vi "Tree_ShowScrollBar.vi"(8 "error in (no error)":errorcluster, 11 "Tree":refnum<vi>) -> (0 "error out":errorcluster)   [LabVIEW 2017]
doc: "Determine, based on the contents of a tree control, whether or not to display its vertical and horizontal scrollbars."
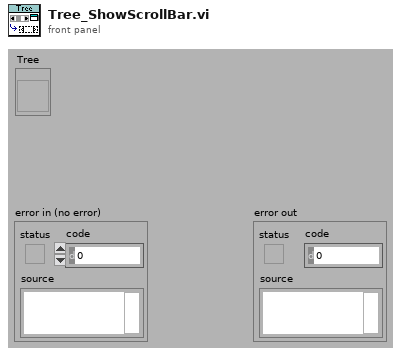
[diagram p1: front panel]
types:
  T1 = enum16{"User-specified Font", "Application Font", "System Font", "Dialog Font"}
  T2 = typedef "LVNodeAndColumnTypeDef.ctl" = cluster{"Node":string, "Column":i32}
  T3 = cluster{"left":i16, "top":i16, "right":i16, "bottom":i16}
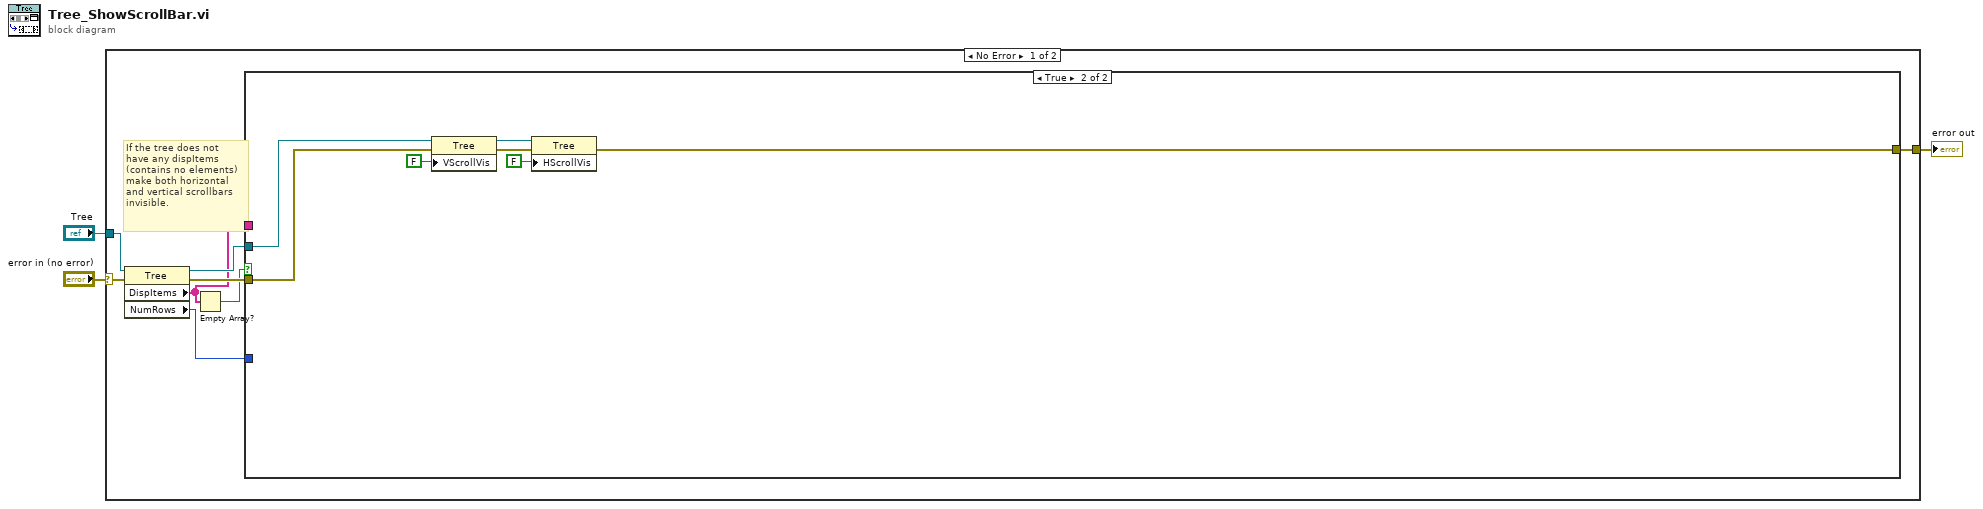
[diagram p0: block diagram]
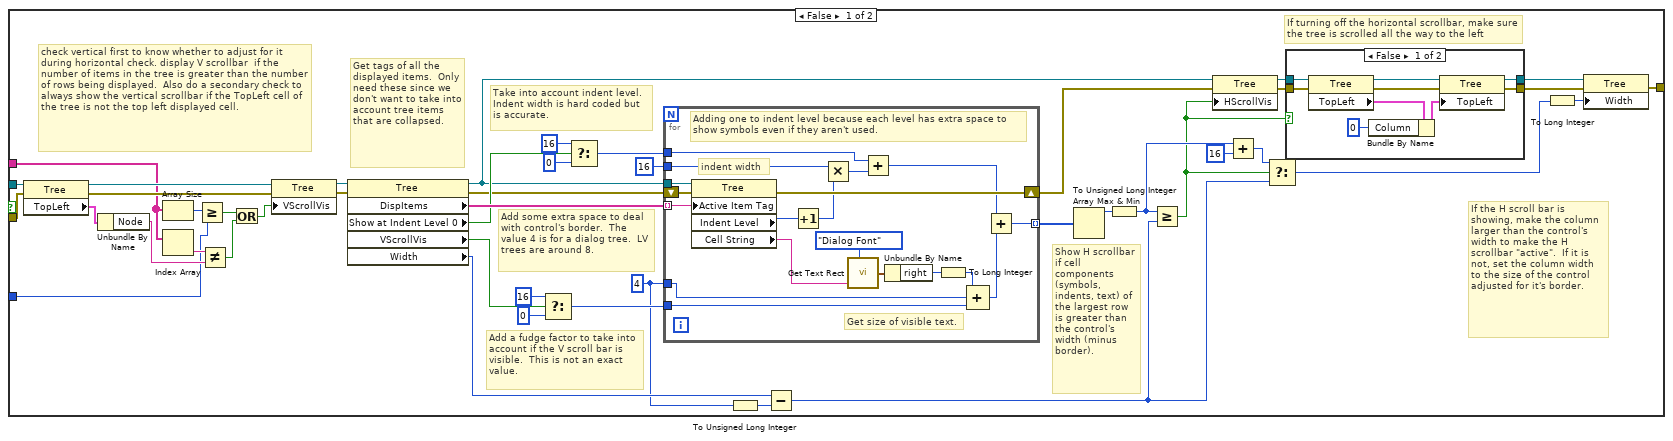
[diagram p2: hidden frame]
diagram:
  n1 = case shown="No Error" "error in (no error)" {
    selector: "error in (no error)" -> [w8 w94]
    tunnel: "Tree" -> [w10 _]
    tunnel: [w11 w94] -> w1
    frame No Error {
      # "If the tree does not\nhave any dispItems\n(contains no elements)\nmake both horizontal\nand vertical scrollbars\ninvisible."
      n2 = property class="Tree"(reference=w10, error in=w8) -> (reference out=w9:refnum<vi>, error out=w7:errorcluster, "DispItems"=w4:string[], "NumRows"=w5:u32)
      n3 = Empty Array?(array=w4) -> (empty?=w6:bool)
      n4 = case shown="True" w6 {
        tunnel: w9 -> [w29 w91]
        tunnel: w7 -> [w28 w90]
        tunnel: [w25 w89] -> w11
        tunnel: w5 -> [w13 _]
        tunnel: w4 -> [w14 _]
        frame False {
          w39 = 4 ("contorl border width")
          # "If turning off the horizontal scrollbar, make sure the tree is scrolled all the way to the left"
          # "check vertical first to know whether to adjust for it during horizontal check. display V scrollbar  if the number of items in the tree is greater than the number of rows being displayed.  Also do a secondary check to always show the vertical scrollbar if the TopLeft cell of the tree is not the top left displayed cell."
          # "If the H scroll bar is showing, make the column larger than the control's width to make the H scrollbar \"active\".  If it is not, set the column width to the size of the control adjusted for it's border."
          # "Show H scrollbar if cell components (symbols, indents, text) of the largest row is greater than  the control's width (minus border)."
          # "Add some extra space to deal with control's border.  The value 4 is for a dialog tree.  LV trees are around 8."
          # "Take into account indent level. Indent width is hard coded but is accurate."
          # "Add a fudge factor to take into account if the V scroll bar is visible.  This is not an exact value."
          # "Get tags of all the displayed items.  Only need these since we don't want to take into account tree items that are collapsed."
          n5 = property class="Tree"(reference=w29, error in=w28) -> (reference out=w32:refnum<vi>, error out=w34:errorcluster, "TopLeft"=w12:T2)
          n6 = Unbundle By Name(w12) -> ("Node"=w21:string)
          n7 = Array Size(array=w14) -> (size(s)=w35:i32)
          n8 = Index Array(array=w14) -> (element=w20:string)  [unwired: 1 in]
          n9 = Greater Or Equal?(x=w35, y=w13) -> (x >= y?=w33:bool)
          n10 = Not Equal?(x=w20, y=w21) -> (x != y?=w22:bool)
          n11 = Or(x=w33, y=w22) -> (x .or. y?=w23:bool)
          n12 = property class="Tree"(reference=w32, error in=w34, "VScrollVis"=w23) -> (reference out=w27:refnum<vi>, error out=w26:errorcluster)
          n13 = property class="Tree"(reference=w27, error in=w26) -> (reference out=w30:refnum<vi>, error out=w31:errorcluster, "DispItems"=w50:string[], "Show at Indent Level 0"=w44:bool, "VScrollVis"=w43:bool, "Width"=w40:u32)
          n14 = Select(t=16 ("y"), s=w43, f=0) -> (s? t:f=w54:i32)
          n15 = Select(t=16 ("y"), s=w44, f=0) -> (s? t:f=w45:i32)
          n16 = for {
            tunnel: w50 -> [w84] mode=indexing
            tunnel: w30 -> [w86]
            tunnel: [w76] -> w51 mode=indexing
            tunnel: w54 -> [w75]
            tunnel: w45 -> [w74]
            tunnel: 16 ("indent width") -> [w73]
            tunnel: w39 -> [w72]
            shift-right: [w71] -> w48
            shift-left: w31 -> [w85]
            # "Adding one to indent level because each level has extra space to show symbols even if they aren't used."
            # "Get size of visible text."
            # "indent width"
            n17 = property class="Tree"(reference=w86, error in=w85, "Active Item Tag"=w84) -> (error out=w71:errorcluster, "Indent Level"=w79:i32, "Cell String"=w80:string)  [unwired: 1 out]
            n18 = Increment(x=w79) -> (x+1=w70:i32)
            n19 = Multiply(x=w73, y=w70) -> (x*y=w78:i32)
            n20 = call <vilib>:"Get Text Rect.vi"("desired font(Application)"=T1."Dialog Font", "text"=w80) -> ("rect"=w82:T3)  [unwired: 4 in, 3 out]
            n21 = Add(x=w74, y=w78) -> (x+y=w68:i32)
            n22 = Unbundle By Name(w82) -> ("right"=w83:i16)
            n23 = To Long Integer(number=w83) -> (32bit integer=w69:i32)
            n24 = Compound Arithmetic op=ADD(w69, w72, w75) -> (w77:i32)
            n25 = Add(x=w68, y=w77) -> (x+y=w76:i32)
          }
          n26 = To Unsigned Long Integer(number=w39) -> (unsigned 32bit integer=w37:u32)
          n27 = Subtract(x=w40, y=w37) -> (x-y=w38:u32)
          n28 = Array Max & Min(array=w51) -> (max value=w55:i32)  [unwired: 3 out]
          n29 = To Unsigned Long Integer(number=w55) -> (unsigned 32bit integer=w36:u32)
          n30 = Greater Or Equal?(x=w36, y=w38) -> (x >= y?=w19:bool)
          n31 = property class="Tree"(reference=w30, error in=w48, "HScrollVis"=w19) -> (reference out=w16:refnum<vi>, error out=w18:errorcluster)
          n32 = Add(x=w36, y=u32 16) -> (x+y=w42:u32)
          n33 = Select(t=w42, s=w19, f=w38) -> (s? t:f=w41:u32)
          n34 = case shown="False" w19 {
            tunnel: w18 -> [w65 w67]
            tunnel: [w60 w67] -> w17
            tunnel: [w63 w66] -> w15
            tunnel: w16 -> [w64 w66]
            frame False {
              n35 = property class="Tree"(reference=w64, error in=w65) -> (reference out=w61:refnum<vi>, error out=w62:errorcluster, "TopLeft"=w59:T2)
              n36 = Bundle By Name(cluster=w59, "Column"=0) -> (w58:T2)
              n37 = property class="Tree"(reference=w61, error in=w62, "TopLeft"=w58) -> (reference out=w63:refnum<vi>, error out=w60:errorcluster)
            }
            frame True {
            }
          }
          n38 = To Long Integer(number=w41) -> (32bit integer=w24:i32)
          n39 = property class="Tree"(reference=w15, error in=w17, "Width"=w24) -> (error out=w25:errorcluster)  [unwired: 1 out]
        }
        frame True {
          n40 = property class="Tree"(reference=w91, error in=w90, "VScrollVis"=FALSE ("Visible Items:Vertical Scrollbar Visible")) -> (reference out=w92:refnum<vi>, error out=w93:errorcluster)
          n41 = property class="Tree"(reference=w92, error in=w93, "HScrollVis"=FALSE ("Visible Items:Horizontal Scrollbar Visible")) -> (error out=w89:errorcluster)  [unwired: 1 out]
        }
      }
    }
    frame Error {
    }
  }
  "error out" <- w1
